vi "LNK CAL CRC 2022-09-02.vi"(11 "Serial number in":string="1000") -> (0 "Loop":i32, 1 "Serial number in Hex":string, 3 "Check SUM HEX":string)   [LabVIEW 2018]
panel:
  out "hex integer string":string
  out "output string (normal display)":string
  out "output string (hex display)":string
  in  "Serial number in Hex 4 Digi":string
  out "Summing of first four bytes BIN":i8 format="%b"
  out "unsigned 16bit integer":u16[](array[numeric])
  # "2022-09-01"
  # "<<<IF 3Digi , Carry =1"
  # "In put Hex 4 Digi here >>>"
  # "<<<< Out put"
  # "Example\nFF FF = 00\nBB AA = 99\n12  FF = ED\n12 12 = DB    **\n11 11 = DD   **\nFF 15 = EA\n\nA2 25 =  38 **\nF7 5D = AA"
  # "11101011"
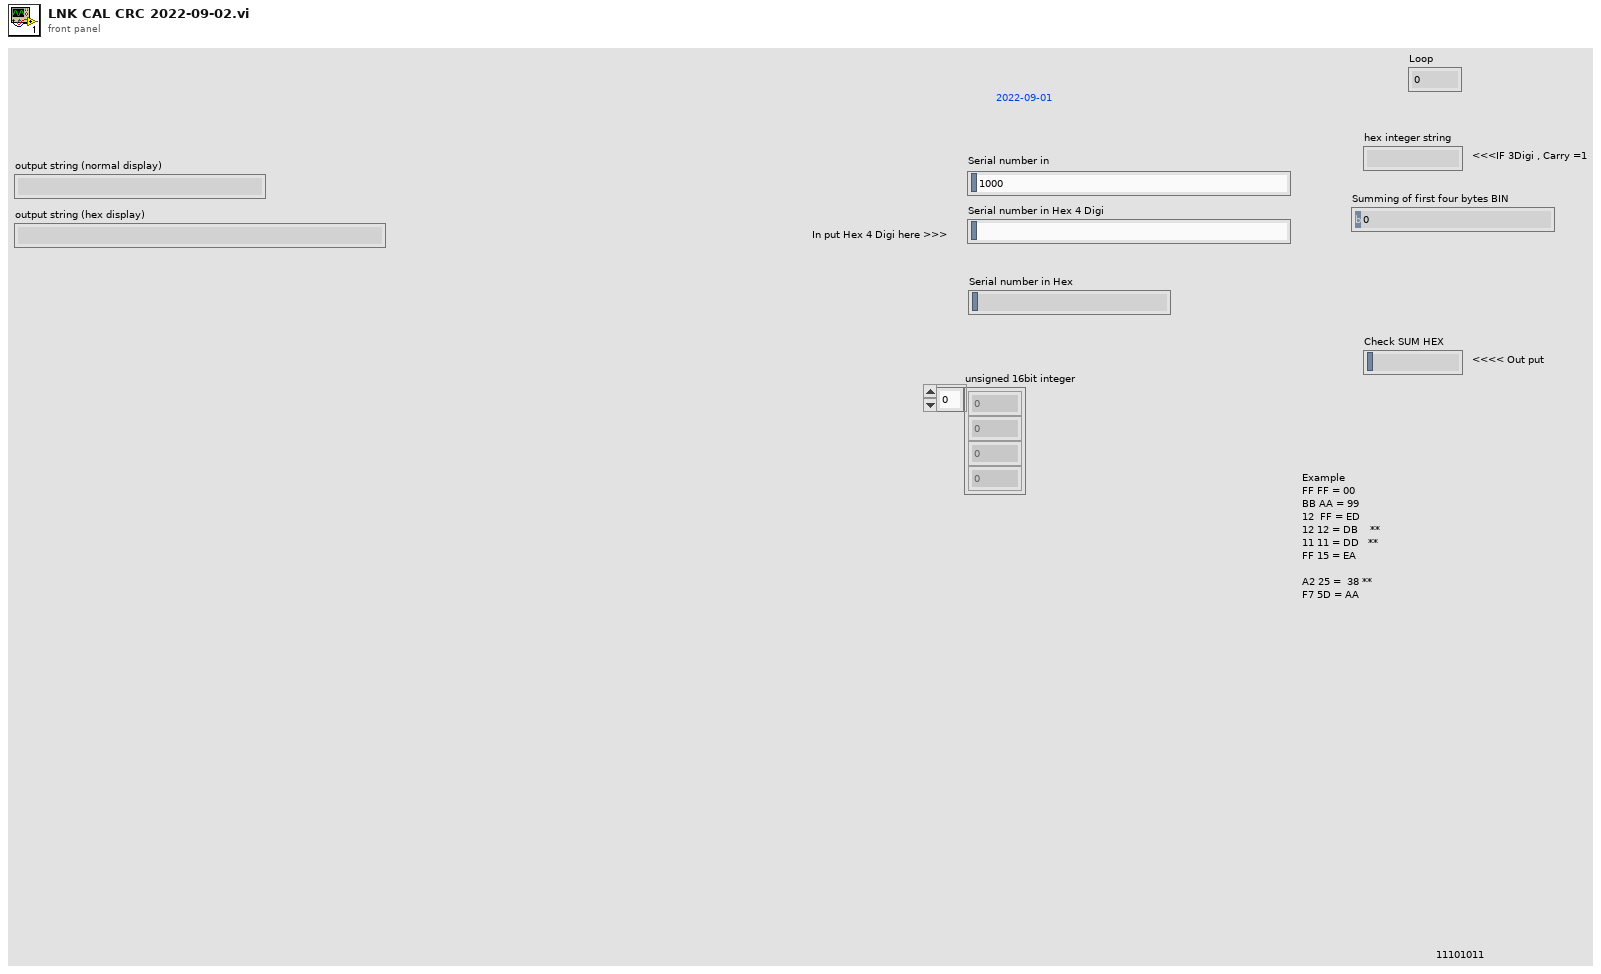
[diagram p1: front panel]
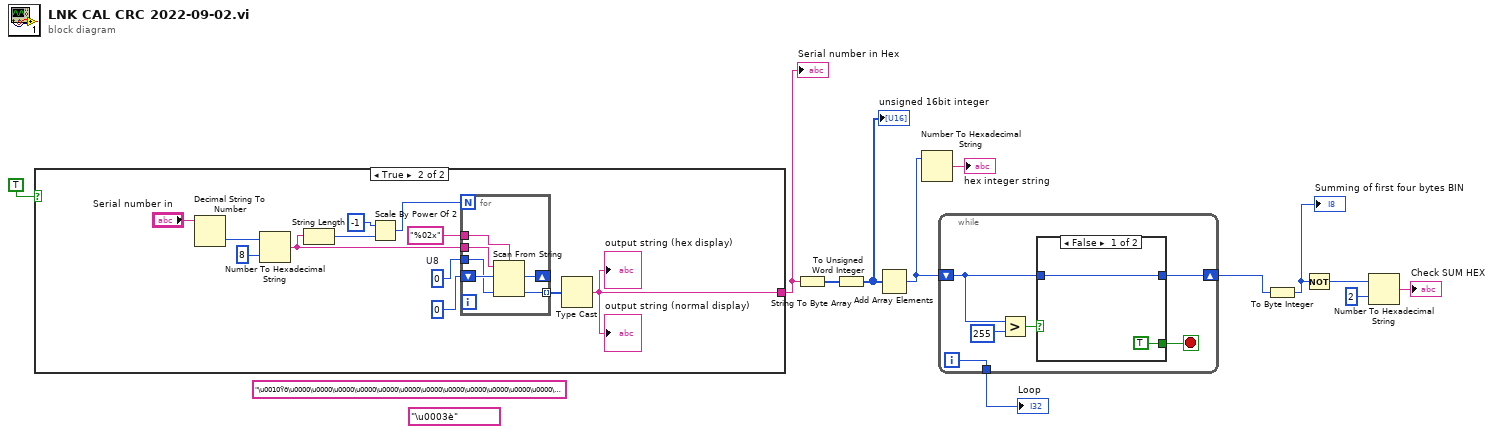
[diagram p0: block diagram]
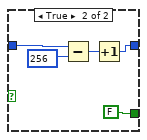
[diagram p2: hidden frame]
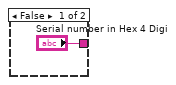
[diagram p3: hidden frame]
diagram:
  (unwired) "\u0003è" ("string")
  (unwired) "\u0010Ÿð\u0000\u0000\u0000\u0000\u0000\u0000\u0000\u0000\u0000\u0000\u0000\u0000\u0000\u0000\u0003è\u0013" ("string")
  n1 = case shown="True" TRUE ("Boolean") {
    tunnel: ["Serial number in Hex 4 Digi" w15] -> w11
    frame False {
    }
    frame True {
      w21 = u8 0  # U8
      n2 = Decimal String To Number(string="Serial number in") -> (number=w25:i32)  [unwired: 2 in, 1 out]
      n3 = Number To Hexadecimal String(1:i16 8 ("width (-)"), 2:w25) -> (0:w14:string)
      n4 = String Length(string=w14) -> (length=w18:i32)
      n5 = Scale By Power Of 2(n=-1, x=w18) -> (x*2^n=w16:i32)
      n6 = for {
        N: w16 -> [_]
        shift-right: [w30] -> _
        shift-left: u32 0 -> [w31]
        tunnel: w14 -> [w29]
        tunnel: w21 -> [w28]
        tunnel: [w27] -> w20 mode=indexing
        tunnel: "%02x" ("format string") -> [w26]
        n7 = Scan From String(format string=w26, input string=w29, initial scan location=w31, default 1=w28) -> (offset past scan=w30:u32, output 1=w27:u8)  [unwired: 1 in, 2 out]
      }
      n8 = Type Cast(x=w20) -> (*(type *) &x=w15:string)  [unwired: 1 in]
      "output string (hex display)" <- w15
      "output string (normal display)" <- w15
    }
  }
  "Serial number in Hex" <- w11
  n9 = String To Byte Array(string=w11) -> (unsigned byte array=w12:u8[])
  n10 = To Unsigned Word Integer(number=w12) -> (unsigned 16bit integer=w9:u16[])
  "unsigned 16bit integer" <- w9
  n11 = Add Array Elements(numeric array=w9) -> (sum=w4:u16)
  n12 = Number To Hexadecimal String(2:w4) -> (0:→"hex integer string":string)  [unwired: 1 in]
  n13 = while {
    shift-right: [w35] -> w3
    shift-left: w4 -> [w34]
    tunnel: [w32] -> w1
    i -> [w32]
    stop <- w33 stop-if-true
    n14 = Greater?(x=w34, y=u16 255) -> (0:w37:bool)
    n15 = case shown="False" w37 {
      tunnel: [w39 w40] -> w35
      tunnel: w34 -> [w39 w43]
      tunnel: [TRUE FALSE] -> w33
      frame False {
      }
      frame True {
        n16 = Subtract(x=w43, y=u16 256) -> (x-y=w41:u16)
        n17 = Increment(x=w41) -> (x+1=w40:u16)
      }
    }
  }
  "Loop" <- w1
  n18 = To Byte Integer(number=w3) -> (8bit integer=w5:i8)
  "Summing of first four bytes BIN" <- w5
  n19 = Not(x=w5) -> (.not. x?=w6:i8)
  n20 = Number To Hexadecimal String(1:i16 2 ("width (-)"), 2:w6) -> (0:→"Check SUM HEX":string)
